vi "SetConfiguration.vi"(8 "error in (no error)":errorcluster, 10 "Configuration":T1={"PhysChan"="SMO-Sim/ai0", "Period (ms)"=50, "input terminal cfg"=-1, "minimum value"=-5.0, "maximum value"=5.0, "units"=enum."Volts", "task name"="", "TDMS File Path"=path "", "Group Name"=""} {"input terminal cfg" items=["Default"=-1, "RSE"=10083, "NRSE"=10078, "Differential"=10106, "Pseudodifferential"=12529]}, 11 "DAQmx-AI":refnum<class "DAQmx-AI.lvclass">) -> (0 "error out":errorcluster, 3 "DAQmx-AI out":refnum<class "DAQmx-AI.lvclass">)   [LabVIEW 2016, in "DAQmx-AI.lvclass"]
doc: "---------------------------------------------------------------\nJKI State Machine Objects™\nhttp://jki.net/state-machine-objects/\nCopyright (C) 2005-2015, JKI <info@jki.net>\nALL RIGHTS RESERVEDJKI State Machine Objects (SMO) 1.0.0.5\nJKI - JKI\nCopyright (c) 2016, JKI"
uses:
  DAQmx-AI.lvclass
  Typedefs/Configuration--Cluster.ctl
  Typedefs/Units -- Enum.ctl
  DAQmx-AI.lvclass/DAQmx-AI.ctl
panel:
  # "For instructions on how to use the JKI State Machine Objects, examples and video tutorials, visit:\nhttp://jki.net/state-machine-objects/\n\nJKI State Machine Objects™\nhttp://jki.net/state-machine-objects/\nCopyright (C) 2005-2015, JKI <info@jki.net>\nALL RIGHTS RESERVED"
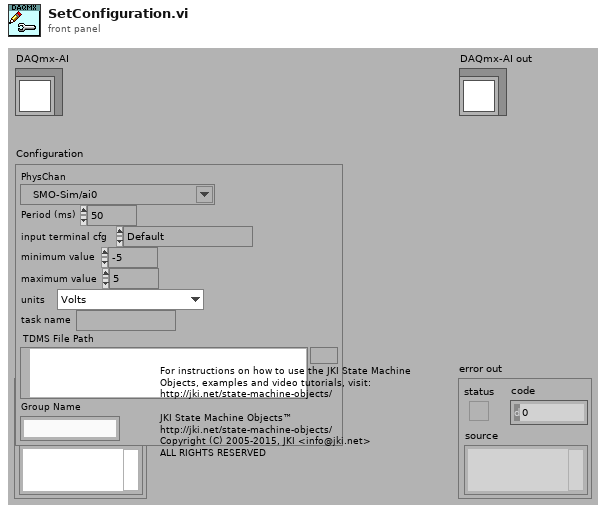
[diagram p1: front panel]
types:
  T1 = typedef "DAQmx-AI.lvclass/Configuration--Cluster.ctl" = cluster{"PhysChan":tag, "Period (ms)":i64, "input terminal cfg":i32, "minimum value":dbl, "maximum value":dbl, "units":T2, "task name":string, "TDMS File Path":path, "Group Name":string}
  T2 = typedef "DAQmx-AI.lvclass/Units -- Enum.ctl" = enum16{"Volts", "Amps", "Deg F", "Deg C", "Deg R", "Kelvins", "Strain", "Ohms", "Hz", "Seconds", "Meters", "Inches", "Degrees", "Radians", "Ticks", "g", "m/s^2", "m/s", "in/s", "Pascals", "Newtons", "Pounds", "kgf", "psi", "bar", "Nm", "oz-in", "lb-in", "lb-ft", "Volts/Volt", "mVolts/Volt", "From TEDS"}
  T3 = typedef "DAQmx-AI.lvclass/PrivateData--Ref.ctl" = refnum<data-value>
  T4 = typedef "DAQmx-AI.lvclass/PrivateData--Cluster.ctl" = cluster{"Configuration":T1, "Public Events":T5, "Data":dbl, "Scaling":T6, "Private Events":T12}
  T5 = typedef "DAQmx-AI.lvclass/PublicEvents--Cluster.ctl" = cluster{"Value Changed":refnum<user-event>, "Task Configuration":refnum<user-event>, "Scaling":refnum<user-event>}
  T6 = typedef "DAQmx-AI.lvclass/Scaling--Cluster.ctl" = cluster{"Scale Name":string, "Scale Type":T7, "Scaled Units":string, "Linear":T8, "Map Range":T9, "Polynomial":T10, "Table":T11}
  T7 = typedef "DAQmx-AI.lvclass/ScalingType--Enum.ctl" = enum16{"No scaling", "Linear", "Map Range", "Polynomial", "Table"}
  T8 = typedef "DAQmx-AI.lvclass/Scaling(Linear)--Cluster.ctl" = cluster{"Slope":dbl, "Intercept":dbl}
  T9 = typedef "DAQmx-AI.lvclass/Scaling(MapRange)--Cluster.ctl" = cluster{"Minimum":dbl, "Maximum":dbl}
  T10 = typedef "DAQmx-AI.lvclass/Scaling(Polynomial)--Cluster.ctl" = cluster{"forward coeff":dbl[], "reverse coeff":dbl[]}
  T11 = typedef "DAQmx-AI.lvclass/Scaling(Table)--Cluster.ctl" = cluster{"scaled values":dbl[], "pres-scaled values":dbl[]}
  T12 = typedef "DAQmx-AI.lvclass/PrivateEvents--Cluster.ctl" = cluster{"Logging":refnum<user-event>}
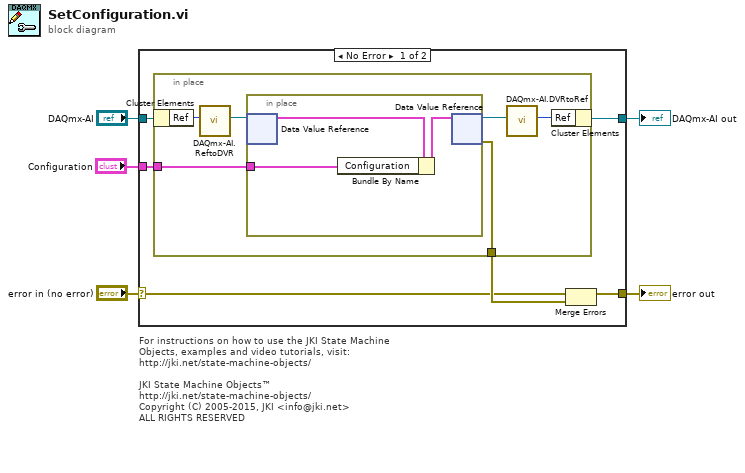
[diagram p0: block diagram]
diagram:
  # "For instructions on how to use the JKI State Machine Objects, examples and video tutorials, visit:\nhttp://jki.net/state-machine-objects/\n\nJKI State Machine Objects™\nhttp://jki.net/state-machine-objects/\nCopyright (C) 2005-2015, JKI <info@jki.net>\nALL RIGHTS RESERVED"
  n1 = case shown="No Error" "error in (no error)" {
    selector: "error in (no error)" -> [w6 w21]
    tunnel: "DAQmx-AI" -> [w7 w22]
    tunnel: [w8 w21] -> w4
    tunnel: [w11 w22] -> w3
    tunnel: "Configuration" -> [w10 _]
    frame No Error {
      n2 = in-place {
        in-place-border: w10 -> [w17]
        in-place-border: [w16] -> w9
        n3 = in-place-cluster #1(w7) -> ("Ref"=w15:u32)
        n4 = call "DAQmx-AI.ReftoDVR.vi"("Ref"=w15) -> ("Ref"=w14:T3)  [unwired: 10 in]
        n5 = in-place {
          in-place-border: w17 -> [w18]
          n6 = in-place-dvr #2(w14) -> (w20:T4)  [unwired: 1 out]
          n7 = Bundle By Name(cluster=w20, "Configuration"=w18) -> (w19:T4)
          n8 = in-place-dvr #2(w19) -> (w13:T3, w16:errorcluster)
        }
        n9 = call "DAQmx-AI.DVRtoRef.vi"("Ref"=w13) -> ("Ref"=w12:u32)  [unwired: 10 in]
        n10 = in-place-cluster #1("Ref"=w12) -> (w11:refnum<class "DAQmx-AI.lvclass">)
      }
      n11 = Merge Errors(w6, w9) -> (w8:errorcluster)
    }
    frame Error {
    }
  }
  "error out" <- w4
  "DAQmx-AI out" <- w3
